vi "VSI Block Write Bytes.vi"(4 "IntervalTime":u32, 5 "BlockNum":u16, 6 "BlockSize":u16, 7 "pWriteData":u8[](array[numeric])=array[10240 elements], 9 "SPIIndex":i32, 10 "DevIndex":i32, 11 "DevType":i32) -> (3 "function return":i32)   [LabVIEW 2010, in "ControlSPI.lvlib"]
doc: "int WINAPI VSI_BlockWriteBytes(int DevType,int DevIndex,int SPIIndex,unsigned char *pWriteData,unsigned short BlockSize,unsigned short BlockNum,unsigned int IntervalTime);"
uses:
  ControlSPI.lvlib
  ControlSPI/Ginkgo_Driver.dll
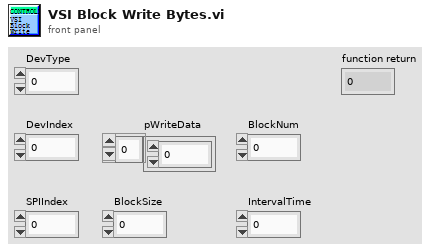
[diagram p1: front panel]
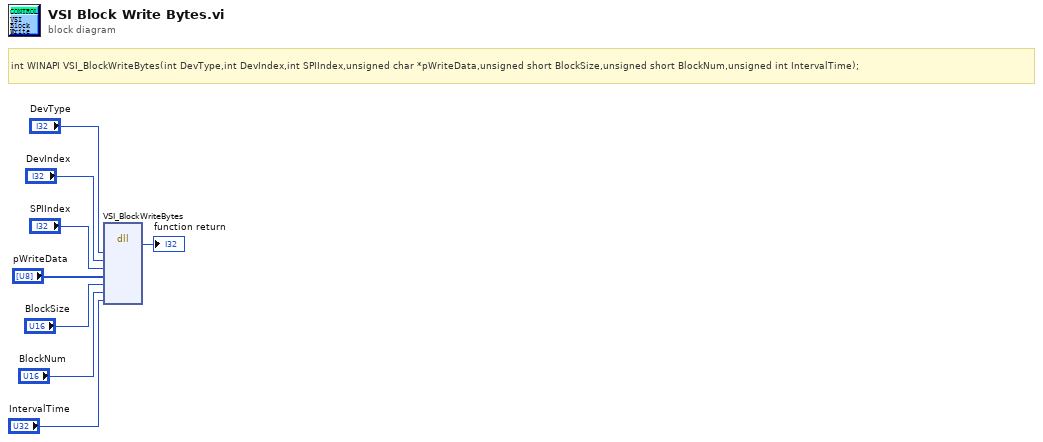
[diagram p0: block diagram]
diagram:
  # "int WINAPI VSI_BlockWriteBytes(int DevType,int DevIndex,int SPIIndex,unsigned char *pWriteData,unsigned short BlockSize,unsigned short BlockNum,unsigned int IntervalTime);"
  n1 = dll-call lib="E:/Project/vt_ginkgo/truck/Ginkgo Driver/vs2010/Ginkgo_USB-I2C&SPI&CAN_API_v2.0.3.3/lib/labview_32bit/ControlSPI/Ginkgo_Driver.*" fn="VSI_BlockWriteBytes"("DevType"="DevType", "DevIndex"="DevIndex", "SPIIndex"="SPIIndex", "pWriteData"="pWriteData", "BlockSize"="BlockSize", "BlockNum"="BlockNum", "IntervalTime"="IntervalTime") -> (→"function return":i32)  [unwired: 10 in, 2 out]
